vi "Restart on Error.vi"(8 "error in (no error)":errorcluster, 10 "Camera error":errorcluster, 11 "Camera Actor in":refnum<class "Camera Actor.lvclass">) -> (0 "error out":errorcluster, 3 "Camera Actor out":refnum<class "Camera Actor.lvclass">)   [LabVIEW 2020, in "Camera Actor.lvlib" / "Camera Actor.lvclass"]
uses:
  Camera Actor.lvclass
  Camera Actor.lvclass/Camera Actor.ctl
  Operation Mode.ctl
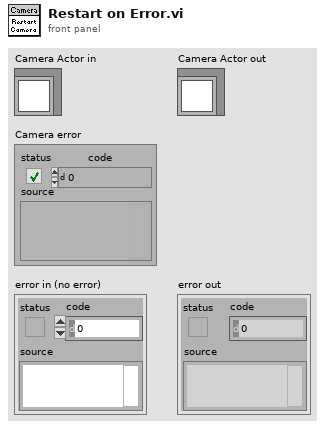
[diagram p1: front panel]
types:
  T1 = typedef "Camera Actor.lvlib/Camera Actor.lvclass/Operation Mode.ctl" = enum16{"Run", "Stop", "Exit", "Error", "Restart"}
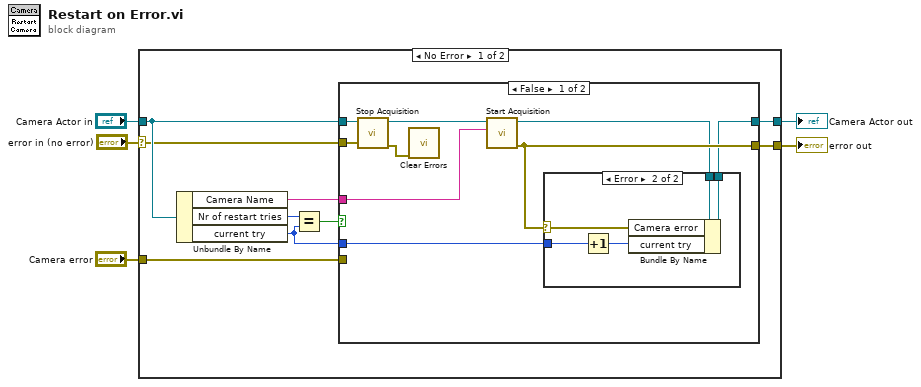
[diagram p0: block diagram]
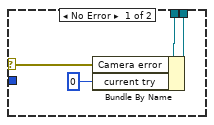
[diagram p2: hidden frame]
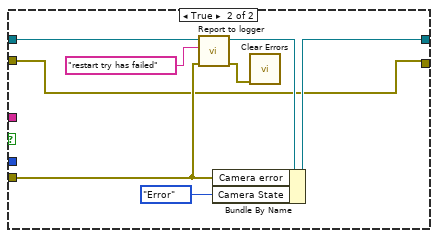
[diagram p3: hidden frame]
diagram:
  n1 = case shown="No Error" "error in (no error)" {
    selector: "error in (no error)" -> [w10 w42]
    tunnel: [w9 w42] -> w4
    tunnel: [w13 w41] -> w2
    tunnel: "Camera Actor in" -> [w12 w41]
    tunnel: "Camera error" -> [w6 _]
    frame No Error {
      n2 = Unbundle By Name(w12) -> ("Camera Name"=w8:string, "Nr of restart tries"=w14:u8, "current try"=w7:u8)
      n3 = Equal?(x=w14, y=w7) -> (x = y?=w11:bool)
      n4 = case shown="False" w11 {
        tunnel: [w16 w39] -> w13
        tunnel: w12 -> [w22 w40]
        tunnel: w10 -> [w20 w35]
        tunnel: [w18 w35] -> w9
        tunnel: w8 -> [w23 _]
        tunnel: w7 -> [w15 _]
        tunnel: w6 -> [_ w36]
        frame False {
          n5 = call-dynamic "Stop Acquisition.vi"("error in (no error)"=w20, "Camera in"=w22) -> ("error out"=w19:errorcluster, "Camera out"=w21:refnum<class "Camera Actor.lvclass">)  [unwired: 8 in]
          n6 = call <vilib>:"Clear Errors.vi"("error in (no error)"=w19) -> ()  [unwired: 5 in, 2 out]
          n7 = call-dynamic "Start Acquisition.vi"("Camera Name"=w23, "Camera in"=w21) -> ("error out"=w18:errorcluster, "Camera out"=w17:refnum<class "Camera Actor.lvclass">)  [unwired: 8 in]
          n8 = case shown="Error" w18 {
            selector: w18 -> [w24 w28]
            tunnel: [w27 w32] -> w16
            tunnel: w17 -> [w25 w31]
            tunnel: w15 -> [_ w30]
            frame No Error {
              n9 = Bundle By Name(cluster=w25, "Camera error"=w24, "current try"=u8 0) -> (w27:refnum<class "Camera Actor.lvclass">)
            }
            frame Error {
              n10 = Increment(x=w30) -> (x+1=w29:u8)
              n11 = Bundle By Name(cluster=w31, "Camera error"=w28, "current try"=w29) -> (w32:refnum<class "Camera Actor.lvclass">)
            }
          }
        }
        frame True {
          n12 = call-dynamic "Report to logger.vi"("error in (no error)"=w36, "Comment"="restart try has failed", "Camera Actor in"=w40) -> ("error out"=w34:errorcluster, "Camera Actor out"=w37:refnum<class "Camera Actor.lvclass">)  [unwired: 7 in]
          n13 = Bundle By Name(cluster=w37, "Camera error"=w36, "Camera State"=Operation_Mode."Error") -> (w39:refnum<class "Camera Actor.lvclass">)
          n14 = call <vilib>:"Clear Errors.vi"("error in (no error)"=w34) -> ()  [unwired: 5 in, 2 out]
        }
      }
    }
    frame Error {
    }
  }
  "error out" <- w4
  "Camera Actor out" <- w2
